vi "PH_Sixpack.set PSDB Axis no Data collection.vi"(0 "i ref in":refnum<vi>, 5 "error in":errorcluster) -> (14 "i ref out":refnum<vi>, 19 "error out":errorcluster)   [LabVIEW 2014]
doc: "This VI sets the PSDB data collection of the axis to \"no data collection\"."
uses:
  PH_Sixpack.lvlib
  PH_Common/PH_PSDB/Data_Status.ctl
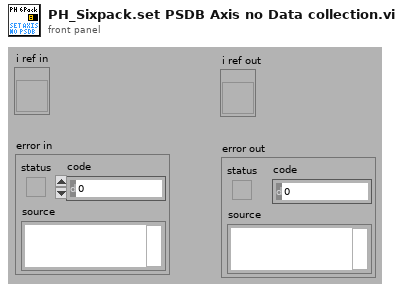
[diagram p1: front panel]
types:
  T1 = typedef "PH_Sixpack.lvlib/PH_Sixpack.i attribute.ctl" = cluster{"Information":cluster{"SixPack ID(0)":u16, "BaudRate(19200)":u16, "COM Port":enum32{"COM1", "COM2", "COM3", "COM4", "COM5", "COM6", "COM7", "COM8", "COM9"}, "HANDLE":i32}, "Serial Number":dbl, "Firmwareversion":dbl, "Axes":T2[], "Status":T6, "Driver Error":errorcluster}
  T2 = typedef "PH_Sixpack.lvlib/PH_Sixpack.MotorCluster.ctl" = cluster{"Wanted 6P Config":cluster{"a max (128)":u16, "V max (300)":u16, "I max % (25)":dbl, "I Power Down (100%)":enum8{"100%", "75%", "50%", "38%", "25%", "19%", "13%", "9%", "0%"}, "I Axis Standing (100%)":enum8{"100%", "75%", "50%", "38%", "25%", "19%", "13%", "9%", "0%"}, "I Const Velocity (100%)":enum8{"100%", "75%", "50%", "38%", "25%", "19%", "13%", "9%", "0%"}, "I Const Accel (100%)":enum8{"100%", "75%", "50%", "38%", "25%", "19%", "13%", "9%", "0%"}, "T Power Down (2)":dbl, "V min (200)":i32, "V start (250)":i32, "Div i (2)":enum8{"0", "1", "2", "3"}, "Poslimit (0)":i32, "P6 Bits":T3, "V ref Max (0)":u16, "Mask for reference \nswitch de-bouncing (0)":u16, "Bit 0 PI Mode (FALSE)":bool, "analog min value (150)":u16, "analog max val (900)":u16, "P5 Bits":T4}, "6P Readout":cluster{"Position":i32, "CurrentActivity":T5, "Analog Input":dbl, "Reference Input":bool}, "Current 6P Config":cluster{"a max (128)":u16, "V max (300)":u16, "I max % (25)":dbl, "I Power Down (100%)":enum8{"100%", "75%", "50%", "38%", "25%", "19%", "13%", "9%", "0%"}, "I Axis Standing (100%)":enum8{"100%", "75%", "50%", "38%", "25%", "19%", "13%", "9%", "0%"}, "I Const Velocity (100%)":enum8{"100%", "75%", "50%", "38%", "25%", "19%", "13%", "9%", "0%"}, "I Const Accel (100%)":enum8{"100%", "75%", "50%", "38%", "25%", "19%", "13%", "9%", "0%"}, "T Power Down (2)":dbl, "V min (200)":i32, "V start (250)":i32, "Div i (2)":enum8{"0", "1", "2", "3"}, "Poslimit (0)":i32, "P6 Bits":T3, "V ref Max (0)":u16, "Mask for reference \nswitch de-bouncing (0)":u16, "Bit 0 PI Mode (FALSE)":bool, "analog min value (150)":u16, "analog max val (900)":u16, "P5 Bits":T4}}
  T3 = typedef "Sixpack.lvlib/MotorParameter_P6.ctl" = cluster{"MT_OPTIMIZEWAY":bool, "MT_FASTREF":bool, "MT_MECHREF":bool, "MT_DELAYTESTNULL":bool, "MT_STOPSOFT":bool, "MT_STOPNOREF":bool, "MT_NULLPOSITIVE":bool, "MUT_STOPFULSTEPS":bool}
  T4 = typedef "Sixpack.lvlib/MotorParameter_P5.ctl" = cluster{"MT_PI":bool, "MT_ROTARY":bool, "MT_AUTONULLCMD":bool, "MT_TESTNULL":bool, "MT_NULLLEFT":bool, "MT_NULLCENTRE":bool, "MT_STOPNULL":bool, "MT_FILTERSWITCH":bool}
  T5 = typedef "Sixpack.lvlib/Activity.ctl" = enum16{"Inactive", "Ramp", "PI-Controller", "Rotation", "ReferenceSearch", "Reference Search", "MechanicalReference"}
  T6 = typedef "PH_Sixpack.Status.ctl" = enum32{"None", "Init", "Configure", "configured", "Close", "closed"}
  T7 = typedef "Data_Status.ctl" = i16
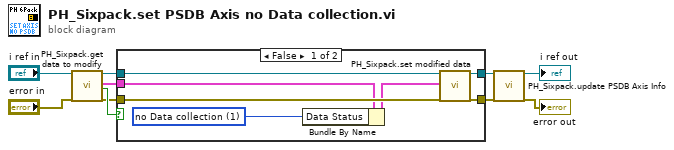
[diagram p0: block diagram]
diagram:
  n1 = call "PH_Sixpack.get data to modify.vi"("i ref in"="i ref in", "error in (no error)"="error in") -> ("i ref out"=w8:refnum<vi>, "i attribute"=w10:T1, "timed out"=w9:bool, "error out"=w6:errorcluster)  [unwired: 14 in]
  n2 = case shown="False" w9 {
    tunnel: w6 -> [w17 w18]
    tunnel: [w11 w18] -> w1
    tunnel: w8 -> [w16 w19]
    tunnel: [w12 w19] -> w3
    tunnel: w10 -> [w15 _]
    frame False {
      w13 = T7 1 items=["no info", "no Data collection", "no problem", "Error getting the instance ID", "Error writing Data to data base", "Error concerning the subsystem", "Error getting the Shot ID", "Error getting the Shot Types", "Error getting the Experiments", "Error verifying wanted Shottype", "Error verifying wanted Experiment"] ("Data Status")
      n3 = Bundle By Name(cluster=w15, "Data Status"=w13) -> (w14:T1)
      n4 = call "PH_Sixpack.set modified data.vi"("i ref in"=w16, "i attribute"=w14, "error in (no error)"=w17) -> ("i ref out"=w12:refnum<vi>, "error out"=w11:errorcluster)  [unwired: 15 in]
    }
    frame True {
    }
  }
  n5 = call "PH_Sixpack.update PSDB Axis Info .vi"("i ref in"=w3, "error in"=w1) -> ("i ref out"=→"i ref out":refnum<vi>, "error out"=→"error out":errorcluster)  [unwired: 16 in]
